vi "ramp_Zstage.vi"(0 "requested z-pos":dbl, 1 "z-pos":dbl, 2 "Move to z":bool) -> ()   [LabVIEW 2020]
uses:
  MotorPosition.vi
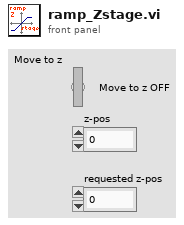
[diagram p1: front panel]
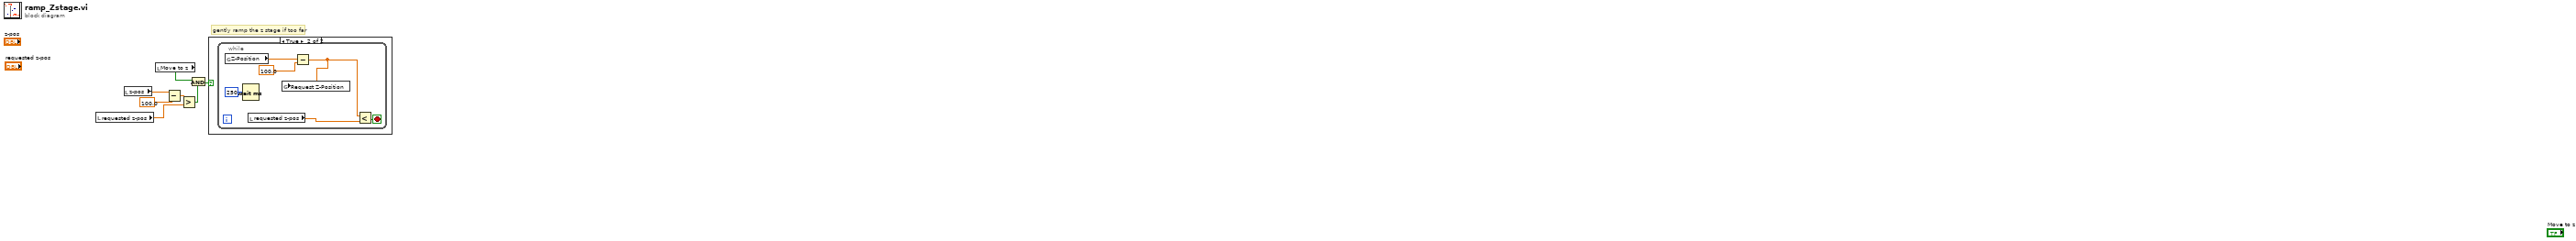
[diagram p0: block diagram]
diagram:
  # "gently ramp the z stage if too far"
  n1 = local read "requested z-pos"() -> (w2:dbl)
  n2 = local read "z-pos"() -> (w4:dbl)
  n3 = local read "Move to z"() -> (w6:bool)
  n4 = Subtract(x=w4, y=100.0) -> (x-y=w3:dbl)
  n5 = Greater?(x=w3, y=w2) -> (0:w1:bool)
  n6 = And(x=w6, y=w1) -> (x .and. y?=w7:bool)
  n7 = case shown="True" w7 {
    frame False {
    }
    frame True {
      n8 = while {
        stop <- w13 stop-if-true
        n9 = global read "MotorPosition.vi" "Z-Position"() -> (w8:dbl)
        n10 = Wait (ms)(milliseconds to wait=u32 250) -> ()  [unwired: 1 out]
        n11 = local read "requested z-pos"() -> (w11:dbl)
        n12 = Subtract(x=w8, y=100.0) -> (x-y=w10:dbl)
        n13 = global write "MotorPosition.vi" "Request Z-Position"(w10) -> ()
        n14 = Less?(x=w10, y=w11) -> (x < y?=w13:bool)
      }
    }
  }
